vi "solar_type Get Value (ASCII).vi"(4 "Boolean as 0,1? (F)":bool, 6 "ArrayDelimiters (1D,2D)":string[](array[string]), 8 "error in (no error)":errorcluster, 9 "Use Enum Names? (F)":bool, 11 "Variant":variant) -> (0 "error out":errorcluster, 2 "Quotes Recommended?":bool, 3 "Value (ASCII)":string)   [LabVIEW 2018]
doc: "This returns the ASCII value of the variant data."
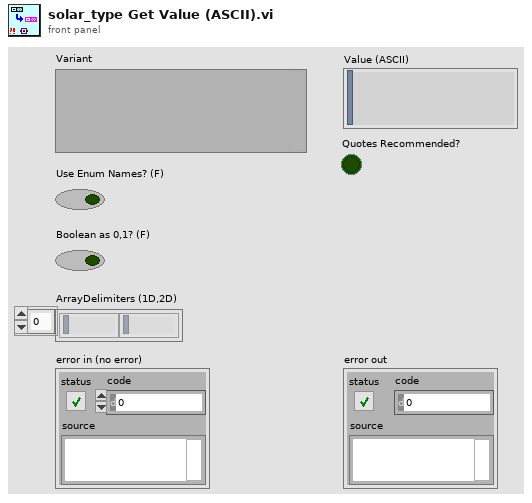
[diagram p1: front panel]
types:
  T1 = typedef "solar_type Item Type.ctl" = enum16{"NULL", "UNKNOWN", "CLUSTER", "I8", "I16", "I32", "I64", "U8", "U16", "U32", "U64", "U8_ENUM", "U16_ENUM", "U32_ENUM", "SGL", "DBL", "BOOLEAN", "STRING", "PATH", "VISA", "TAG", "TIME", "I8_1D", "I16_1D", "I32_1D", "I64_1D", "U8_1D", "U16_1D", "U32_1D", "U64_1D", "U8_ENUM_1D", "U16_ENUM_1D", "U32_ENUM_1D", "SGL_1D", "DBL_1D", "BOOLEAN_1D", "STRING_1D", "PATH_1D", "VISA_1D", "TAG_1D", "TIME_1D", "I8_2D", "I16_2D", "I32_2D", "I64_2D", "U8_2D", "U16_2D", "U32_2D", "U64_2D", "U8_ENUM_2D", "U16_ENUM_2D", "U32_ENUM_2D", "SGL_2D", "DBL_2D", "BOOLEAN_2D", "STRING_2D", "PATH_2D", "VISA_2D", "TAG_2D", "TIME_2D"}
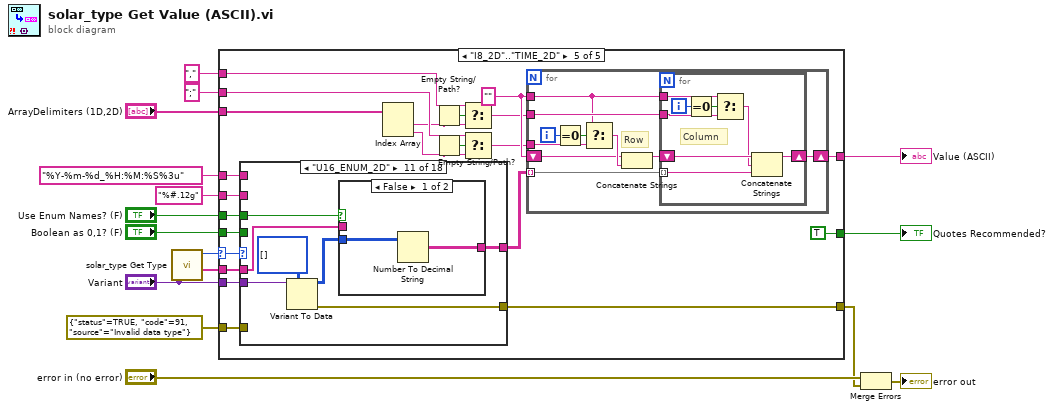
[diagram p0: block diagram]
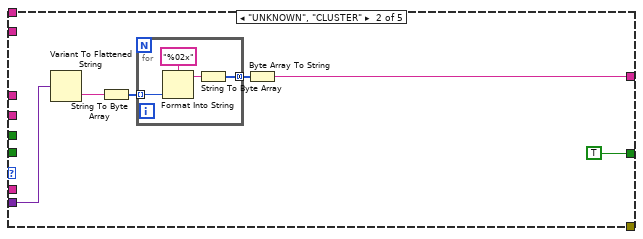
[diagram p3: hidden frame]
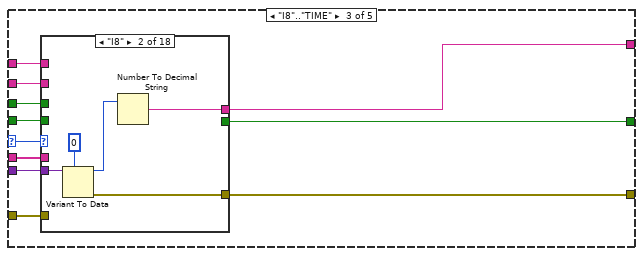
[diagram p4: hidden frame]
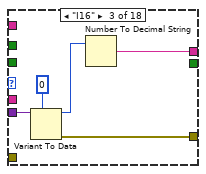
[diagram p6: hidden frame]
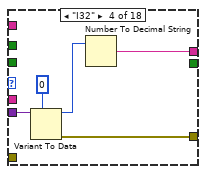
[diagram p7: hidden frame]
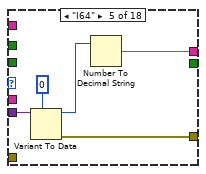
[diagram p8: hidden frame]
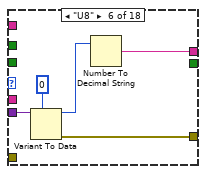
[diagram p9: hidden frame]
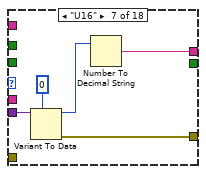
[diagram p10: hidden frame]
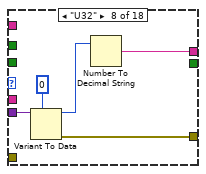
[diagram p11: hidden frame]
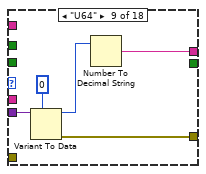
[diagram p12: hidden frame]
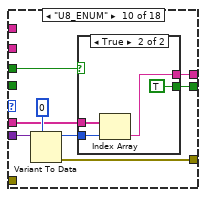
[diagram p13: hidden frame]
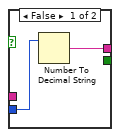
[diagram p14: hidden frame]
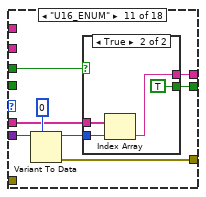
[diagram p15: hidden frame]
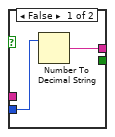
[diagram p16: hidden frame]
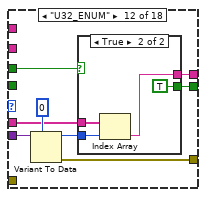
[diagram p17: hidden frame]
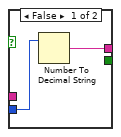
[diagram p18: hidden frame]
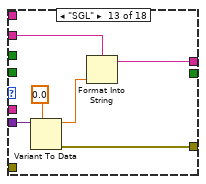
[diagram p19: hidden frame]
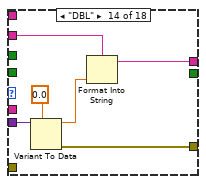
[diagram p20: hidden frame]
diagram:
  n1 = call "solar_type Get Type.vi"("Variant"="Variant") -> ("Type"=w8:T1, "Enum Names"=w2:string[])  [unwired: 4 in, 1 out]
  n2 = case shown="\"I8_2D\"..\"TIME_2D\"" w8 {
    selector: w8 -> [_ _ w36 w177 w347]
    tunnel: "Variant" -> [_ w20 w38 w178 w349]
    tunnel: [_ w21 w34 w181 w345] -> w13
    tunnel: "%Y-%m-%d_%H:%M:%S%3u" -> [_ _ w32 w173 w341]
    tunnel: [w17 _ w37 w175 w348] -> w6
    tunnel: errorcluster {"status"=TRUE, "code"=91, "source"="Invalid data type"} ("error in (no error)") -> [w17 _ w35 w179 w346]
    tunnel: "%#.12g" ("format string") -> [_ _ w33 w174 w342]
    tunnel: "," -> [_ _ _ w170 w336]
    tunnel: ";" -> [_ _ _ _ w335]
    tunnel: "Boolean as 0,1? (F)" -> [_ _ w31 w169 w334]
    tunnel: "ArrayDelimiters (1D,2D)" -> [_ _ _ w168 w333]
    tunnel: "Use Enum Names? (F)" -> [_ _ w30 w166 w330]
    tunnel: w2 -> [_ _ w29 w165 w329]
    tunnel: [_ TRUE w28 TRUE TRUE] -> w1
    frame "NULL" {
    }
    frame "UNKNOWN", "CLUSTER" {
      n3 = Variant To Flattened String(Variant=w20) -> (data string=w19:string)  [unwired: 1 out]
      n4 = String To Byte Array(string=w19) -> (unsigned byte array=w23:u8[])
      n5 = for {
        tunnel: w23 -> [w27] mode=indexing
        tunnel: [w24] -> w22 mode=concatenating
        n6 = Format Into String(format string="%02x" ("Format String"), w27) -> (resulting string=w25:string)  [unwired: 2 in, 1 out]
        n7 = String To Byte Array(string=w25) -> (unsigned byte array=w24:u8[])
      }
      n8 = Byte Array To String(unsigned byte array=w22) -> (string=w21:string)
    }
    frame "I8".."TIME" {
      n9 = case shown="\"I8\"" w36 {
        tunnel: w38 -> [_ w44 w49 w54 w59 w64 w69 w74 w79 w87 w101 w115 w127 w133 w145 w150 w156 w163]
        tunnel: [w39 w43 w48 w53 w58 w63 w68 w73 w78 w86 w100 w114 w126 w132 w144 w149 w155 w162] -> w37
        tunnel: w35 -> [w39 _ _ _ _ _ _ _ _ _ _ _ _ _ _ _ _ _]
        tunnel: [_ w40 w45 w50 w55 w60 w65 w70 w75 w83 w96 w109 w123 w129 w141 w147 w152 w159] -> w34
        tunnel: w33 -> [_ _ _ _ _ _ _ _ _ _ _ _ w122 w128 _ _ _ _]
        tunnel: w32 -> [_ _ _ _ _ _ _ _ _ _ _ _ _ _ _ _ _ w158]
        tunnel: w31 -> [_ _ _ _ _ _ _ _ _ _ _ _ _ _ w136 _ _ _]
        tunnel: w30 -> [_ _ _ _ _ _ _ _ _ w81 w95 w110 _ _ _ _ _ _]
        tunnel: w29 -> [_ _ _ _ _ _ _ _ _ w84 w98 w112 _ _ _ _ _ _]
        tunnel: [_ _ _ _ _ _ _ _ _ w80 w94 w108 _ _ _ TRUE TRUE TRUE] -> w28
        frame "NULL".."CLUSTER", "I8_1D".."TIME_2D" {
        }
        frame "I8" {
          n10 = Variant To Data(type=i8 0, Variant=w44) -> (data=w41:i8, error out=w43:errorcluster)  [unwired: 1 in]
          n11 = Number To Decimal String(number=w41) -> (decimal integer string=w40:string)  [unwired: 1 in]
        }
        frame "I16" {
          n12 = Variant To Data(type=i16 0, Variant=w49) -> (data=w46:i16, error out=w48:errorcluster)  [unwired: 1 in]
          n13 = Number To Decimal String(number=w46) -> (decimal integer string=w45:string)  [unwired: 1 in]
        }
        frame "I32" {
          n14 = Variant To Data(type=0, Variant=w54) -> (data=w51:i32, error out=w53:errorcluster)  [unwired: 1 in]
          n15 = Number To Decimal String(number=w51) -> (decimal integer string=w50:string)  [unwired: 1 in]
        }
        frame "I64" {
          n16 = Variant To Data(type=i64 0, Variant=w59) -> (data=w56:i64, error out=w58:errorcluster)  [unwired: 1 in]
          n17 = Number To Decimal String(number=w56) -> (decimal integer string=w55:string)  [unwired: 1 in]
        }
        frame "U8" {
          n18 = Variant To Data(type=u8 0, Variant=w64) -> (data=w61:u8, error out=w63:errorcluster)  [unwired: 1 in]
          n19 = Number To Decimal String(number=w61) -> (decimal integer string=w60:string)  [unwired: 1 in]
        }
        frame "U16" {
          n20 = Variant To Data(type=u16 0, Variant=w69) -> (data=w66:u16, error out=w68:errorcluster)  [unwired: 1 in]
          n21 = Number To Decimal String(number=w66) -> (decimal integer string=w65:string)  [unwired: 1 in]
        }
        frame "U32" {
          n22 = Variant To Data(type=u32 0, Variant=w74) -> (data=w71:u32, error out=w73:errorcluster)  [unwired: 1 in]
          n23 = Number To Decimal String(number=w71) -> (decimal integer string=w70:string)  [unwired: 1 in]
        }
        frame "U64" {
          n24 = Variant To Data(type=u64 0, Variant=w79) -> (data=w76:u64, error out=w78:errorcluster)  [unwired: 1 in]
          n25 = Number To Decimal String(number=w76) -> (decimal integer string=w75:string)  [unwired: 1 in]
        }
        frame "U8_ENUM" {
          n26 = Variant To Data(type=u8 0, Variant=w87) -> (data=w82:u8, error out=w86:errorcluster)  [unwired: 1 in]
          n27 = case shown="True" w81 {
            tunnel: w84 -> [_ w93]
            tunnel: [w88 w92] -> w83
            tunnel: w82 -> [w89 w91]
            tunnel: [_ TRUE] -> w80
            frame False {
              n28 = Number To Decimal String(number=w89) -> (decimal integer string=w88:string)  [unwired: 1 in]
            }
            frame True {
              n29 = Index Array(array=w93, index=w91) -> (element=w92:string)
            }
          }
        }
        frame "U16_ENUM" {
          n30 = Variant To Data(type=u16 0, Variant=w101) -> (data=w97:u16, error out=w100:errorcluster)  [unwired: 1 in]
          n31 = case shown="True" w95 {
            tunnel: w98 -> [_ w107]
            tunnel: [w102 w106] -> w96
            tunnel: w97 -> [w103 w105]
            tunnel: [_ TRUE] -> w94
            frame False {
              n32 = Number To Decimal String(number=w103) -> (decimal integer string=w102:string)  [unwired: 1 in]
            }
            frame True {
              n33 = Index Array(array=w107, index=w105) -> (element=w106:string)
            }
          }
        }
        frame "U32_ENUM" {
          n34 = Variant To Data(type=u32 0, Variant=w115) -> (data=w111:u32, error out=w114:errorcluster)  [unwired: 1 in]
          n35 = case shown="True" w110 {
            tunnel: w112 -> [_ w121]
            tunnel: [w116 w120] -> w109
            tunnel: w111 -> [w117 w119]
            tunnel: [_ TRUE] -> w108
            frame False {
              n36 = Number To Decimal String(number=w117) -> (decimal integer string=w116:string)  [unwired: 1 in]
            }
            frame True {
              n37 = Index Array(array=w121, index=w119) -> (element=w120:string)
            }
          }
        }
        frame "SGL" {
          n38 = Variant To Data(type=sgl 0.0, Variant=w127) -> (data=w124:sgl, error out=w126:errorcluster)  [unwired: 1 in]
          n39 = Format Into String(format string=w122, w124) -> (resulting string=w123:string)  [unwired: 2 in, 1 out]
        }
        frame "DBL" {
          n40 = Variant To Data(type=0.0, Variant=w133) -> (data=w130:dbl, error out=w132:errorcluster)  [unwired: 1 in]
          n41 = Format Into String(format string=w128, w130) -> (resulting string=w129:string)  [unwired: 2 in, 1 out]
        }
        frame "BOOLEAN" {
          n42 = Variant To Data(type=FALSE, Variant=w145) -> (data=w142:bool, error out=w144:errorcluster)  [unwired: 1 in]
          n43 = Select(t="1", s=w136, f="true") -> (s? t:f=w135:string)
          n44 = Select(t="0", s=w136, f="false") -> (s? t:f=w134:string)
          n45 = Select(t=w135, s=w142, f=w134) -> (s? t:f=w141:string)
        }
        frame "STRING", "VISA", "TAG" {
          n46 = Variant To Data(type="", Variant=w150) -> (data=w147:string, error out=w149:errorcluster)  [unwired: 1 in]
        }
        frame "PATH" {
          n47 = Variant To Data(type=path "", Variant=w156) -> (data=w153:path, error out=w155:errorcluster)  [unwired: 1 in]
          n48 = Path To String(path=w153) -> (string=w152:string)
        }
        frame "TIME" {
          n49 = Variant To Data(type=timestamp(0 s since 1904-01-01), Variant=w163) -> (data=w160:timestamp, error out=w162:errorcluster)  [unwired: 1 in]
          n50 = Format Date/Time String(time format string (%c)=w158, seconds (now)=w160) -> (date/time string=w159:string)  [unwired: 1 in]
        }
      }
    }
    frame "I8_1D".."TIME_1D" {
      w180 = ""
      n51 = case shown="\"U8_ENUM_1D\"" w177 {
        tunnel: w178 -> [_ w187 w192 w197 w202 w207 w212 w217 w222 w229 w244 w259 w273 w282 w297 w305 w310 w316]
        tunnel: [w182 w186 w191 w196 w201 w206 w211 w216 w221 w228 w243 w258 w272 w281 w296 w304 w309 w315] -> w175
        tunnel: w179 -> [w182 _ _ _ _ _ _ _ _ _ _ _ _ _ _ _ _ _]
        tunnel: [_ w183 w188 w193 w198 w203 w208 w213 w218 w224 w239 w254 w269 w278 w293 w302 w306 w312] -> w176
        tunnel: w174 -> [_ _ _ _ _ _ _ _ _ _ _ _ w268 w277 _ _ _ _]
        tunnel: w173 -> [_ _ _ _ _ _ _ _ _ _ _ _ _ _ _ _ _ w311]
        tunnel: w169 -> [_ _ _ _ _ _ _ _ _ _ _ _ _ _ w288 _ _ _]
        tunnel: w166 -> [_ _ _ _ _ _ _ _ _ w225 w240 w255 _ _ _ _ _ _]
        tunnel: w165 -> [_ _ _ _ _ _ _ _ _ w223 w238 w253 _ _ _ _ _ _]
        frame "NULL".."TIME", "I8_2D".."TIME_2D" {
        }
        frame "I8_1D" {
          n52 = Variant To Data(type=i8[] [], Variant=w187) -> (data=w184:i8[], error out=w186:errorcluster)  [unwired: 1 in]
          n53 = Number To Decimal String(number=w184) -> (decimal integer string=w183:string[])  [unwired: 1 in]
        }
        frame "I16_1D" {
          n54 = Variant To Data(type=i16[] [], Variant=w192) -> (data=w189:i16[], error out=w191:errorcluster)  [unwired: 1 in]
          n55 = Number To Decimal String(number=w189) -> (decimal integer string=w188:string[])  [unwired: 1 in]
        }
        frame "I32_1D" {
          n56 = Variant To Data(type=i32[] [], Variant=w197) -> (data=w194:i32[], error out=w196:errorcluster)  [unwired: 1 in]
          n57 = Number To Decimal String(number=w194) -> (decimal integer string=w193:string[])  [unwired: 1 in]
        }
        frame "I64_1D" {
          n58 = Variant To Data(type=i64[] [], Variant=w202) -> (data=w199:i64[], error out=w201:errorcluster)  [unwired: 1 in]
          n59 = Number To Decimal String(number=w199) -> (decimal integer string=w198:string[])  [unwired: 1 in]
        }
        frame "U8_1D" {
          n60 = Variant To Data(type=u8[] [], Variant=w207) -> (data=w204:u8[], error out=w206:errorcluster)  [unwired: 1 in]
          n61 = Number To Decimal String(number=w204) -> (decimal integer string=w203:string[])  [unwired: 1 in]
        }
        frame "U16_1D" {
          n62 = Variant To Data(type=u16[] [], Variant=w212) -> (data=w209:u16[], error out=w211:errorcluster)  [unwired: 1 in]
          n63 = Number To Decimal String(number=w209) -> (decimal integer string=w208:string[])  [unwired: 1 in]
        }
        frame "U32_1D" {
          n64 = Variant To Data(type=u32[] [], Variant=w217) -> (data=w214:u32[], error out=w216:errorcluster)  [unwired: 1 in]
          n65 = Number To Decimal String(number=w214) -> (decimal integer string=w213:string[])  [unwired: 1 in]
        }
        frame "U64_1D" {
          n66 = Variant To Data(type=u64[] [], Variant=w222) -> (data=w219:u64[], error out=w221:errorcluster)  [unwired: 1 in]
          n67 = Number To Decimal String(number=w219) -> (decimal integer string=w218:string[])  [unwired: 1 in]
        }
        frame "U8_ENUM_1D" {
          n68 = Variant To Data(type=u8[] [], Variant=w229) -> (data=w226:u8[], error out=w228:errorcluster)  [unwired: 1 in]
          n69 = case shown="True" w225 {
            tunnel: w223 -> [_ w234]
            tunnel: [w230 w233] -> w224
            tunnel: w226 -> [w231 w232]
            frame False {
              n70 = Number To Decimal String(number=w231) -> (decimal integer string=w230:string[])  [unwired: 1 in]
            }
            frame True {
              n71 = for {
                tunnel: w234 -> [w237]
                tunnel: [w236] -> w233 mode=indexing
                tunnel: w232 -> [w235] mode=indexing
                n72 = Index Array(array=w237, index=w235) -> (element=w236:string)
              }
            }
          }
        }
        frame "U16_ENUM_1D" {
          n73 = Variant To Data(type=u16[] [], Variant=w244) -> (data=w241:u16[], error out=w243:errorcluster)  [unwired: 1 in]
          n74 = case shown="True" w240 {
            tunnel: w238 -> [_ w249]
            tunnel: [w245 w248] -> w239
            tunnel: w241 -> [w246 w247]
            frame False {
              n75 = Number To Decimal String(number=w246) -> (decimal integer string=w245:string[])  [unwired: 1 in]
            }
            frame True {
              n76 = for {
                tunnel: w249 -> [w252]
                tunnel: [w251] -> w248 mode=indexing
                tunnel: w247 -> [w250] mode=indexing
                n77 = Index Array(array=w252, index=w250) -> (element=w251:string)
              }
            }
          }
        }
        frame "U32_ENUM_1D" {
          n78 = Variant To Data(type=u32[] [], Variant=w259) -> (data=w256:u32[], error out=w258:errorcluster)  [unwired: 1 in]
          n79 = case shown="True" w255 {
            tunnel: w253 -> [_ w264]
            tunnel: [w260 w263] -> w254
            tunnel: w256 -> [w261 w262]
            frame False {
              n80 = Number To Decimal String(number=w261) -> (decimal integer string=w260:string[])  [unwired: 1 in]
            }
            frame True {
              n81 = for {
                tunnel: w264 -> [w267]
                tunnel: [w266] -> w263 mode=indexing
                tunnel: w262 -> [w265] mode=indexing
                n82 = Index Array(array=w267, index=w265) -> (element=w266:string)
              }
            }
          }
        }
        frame "SGL_1D" {
          n83 = Variant To Data(type=sgl[] [], Variant=w273) -> (data=w270:sgl[], error out=w272:errorcluster)  [unwired: 1 in]
          n84 = for {
            tunnel: w270 -> [w276] mode=indexing
            tunnel: [w275] -> w269 mode=indexing
            tunnel: w268 -> [w274]
            n85 = Format Into String(format string=w274, w276) -> (resulting string=w275:string)  [unwired: 2 in, 1 out]
          }
        }
        frame "DBL_1D" {
          n86 = Variant To Data(type=dbl[] [], Variant=w282) -> (data=w279:dbl[], error out=w281:errorcluster)  [unwired: 1 in]
          n87 = for {
            tunnel: w279 -> [w285] mode=indexing
            tunnel: [w284] -> w278 mode=indexing
            tunnel: w277 -> [w283]
            n88 = Format Into String(format string=w283, w285) -> (resulting string=w284:string)  [unwired: 2 in, 1 out]
          }
        }
        frame "BOOLEAN_1D" {
          n89 = Variant To Data(type=bool[] [], Variant=w297) -> (data=w294:bool[], error out=w296:errorcluster)  [unwired: 1 in]
          n90 = Select(t="1", s=w288, f="true") -> (s? t:f=w287:string)
          n91 = Select(t="0", s=w288, f="false") -> (s? t:f=w286:string)
          n92 = for {
            tunnel: w294 -> [w301] mode=indexing
            tunnel: [w300] -> w293 mode=indexing
            tunnel: w287 -> [w299]
            tunnel: w286 -> [w298]
            n93 = Select(t=w299, s=w301, f=w298) -> (s? t:f=w300:string)
          }
        }
        frame "STRING_1D", "VISA_1D", "TAG_1D" {
          n94 = Variant To Data(type=string[] [], Variant=w305) -> (data=w302:string[], error out=w304:errorcluster)  [unwired: 1 in]
        }
        frame "PATH_1D" {
          n95 = Variant To Data(type=path[] [], Variant=w310) -> (data=w307:path[], error out=w309:errorcluster)  [unwired: 1 in]
          n96 = Path To String(path=w307) -> (string=w306:string[])
        }
        frame "TIME_1D" {
          n97 = Variant To Data(type=timestamp[] [], Variant=w316) -> (data=w313:timestamp[], error out=w315:errorcluster)  [unwired: 1 in]
          n98 = for {
            tunnel: w313 -> [w317] mode=indexing
            tunnel: [w319] -> w312 mode=indexing
            tunnel: w311 -> [w318]
            n99 = Format Date/Time String(time format string (%c)=w318, seconds (now)=w317) -> (date/time string=w319:string)  [unwired: 1 in]
          }
        }
      }
      n100 = Index Array(array=w168) -> (element=w167:string)  [unwired: 1 in]
      n101 = Empty String/Path?(string/path=w167) -> (empty?=w172:bool)
      n102 = Select(t=w170, s=w172, f=w167) -> (s? t:f=w171:string)
      n103 = for {
        shift-right: [w326] -> w181
        shift-left: w180 -> [w327]
        tunnel: w171 -> [w322]
        tunnel: w180 -> [w321]
        tunnel: w176 -> [w320] mode=indexing
        i -> [w325]
        # "Column"
        n104 = Equal To 0?(x=w325) -> (x = 0?=w324:bool)
        n105 = Select(t=w321, s=w324, f=w322) -> (s? t:f=w323:string)
        n106 = Concatenate Strings(w327, w323, w320) -> (w326:string)
      }
    }
    frame "I8_2D".."TIME_2D" {
      w344 = ""
      n107 = case shown="\"U16_ENUM_2D\"" w347 {
        tunnel: w349 -> [_ w355 w360 w365 w370 w375 w380 w385 w390 w397 w415 w433 w450 w462 w480 w492 w497 w503]
        tunnel: [w350 w354 w359 w364 w369 w374 w379 w384 w389 w396 w414 w432 w449 w461 w479 w491 w496 w502] -> w348
        tunnel: w346 -> [w350 _ _ _ _ _ _ _ _ _ _ _ _ _ _ _ _ _]
        tunnel: [_ w351 w356 w361 w366 w371 w376 w381 w386 w391 w409 w427 w446 w458 w477 w489 w493 w499] -> w343
        tunnel: w342 -> [_ _ _ _ _ _ _ _ _ _ _ _ w445 w457 _ _ _ _]
        tunnel: w341 -> [_ _ _ _ _ _ _ _ _ _ _ _ _ _ _ _ _ w498]
        tunnel: w334 -> [_ _ _ _ _ _ _ _ _ _ _ _ _ _ w471 _ _ _]
        tunnel: w330 -> [_ _ _ _ _ _ _ _ _ w393 w411 w429 _ _ _ _ _ _]
        tunnel: w329 -> [_ _ _ _ _ _ _ _ _ w392 w410 w428 _ _ _ _ _ _]
        frame "NULL".."TIME_1D" {
        }
        frame "I8_2D" {
          n108 = Variant To Data(type=i8[][] [], Variant=w355) -> (data=w352:i8[][], error out=w354:errorcluster)  [unwired: 1 in]
          n109 = Number To Decimal String(number=w352) -> (decimal integer string=w351:string[][])  [unwired: 1 in]
        }
        frame "I16_2D" {
          n110 = Variant To Data(type=i16[][] [], Variant=w360) -> (data=w357:i16[][], error out=w359:errorcluster)  [unwired: 1 in]
          n111 = Number To Decimal String(number=w357) -> (decimal integer string=w356:string[][])  [unwired: 1 in]
        }
        frame "I32_2D" {
          n112 = Variant To Data(type=i32[][] [], Variant=w365) -> (data=w362:i32[][], error out=w364:errorcluster)  [unwired: 1 in]
          n113 = Number To Decimal String(number=w362) -> (decimal integer string=w361:string[][])  [unwired: 1 in]
        }
        frame "I64_2D" {
          n114 = Variant To Data(type=i64[][] [], Variant=w370) -> (data=w367:i64[][], error out=w369:errorcluster)  [unwired: 1 in]
          n115 = Number To Decimal String(number=w367) -> (decimal integer string=w366:string[][])  [unwired: 1 in]
        }
        frame "U8_2D" {
          n116 = Variant To Data(type=u8[][] [], Variant=w375) -> (data=w372:u8[][], error out=w374:errorcluster)  [unwired: 1 in]
          n117 = Number To Decimal String(number=w372) -> (decimal integer string=w371:string[][])  [unwired: 1 in]
        }
        frame "U16_2D" {
          n118 = Variant To Data(type=u16[][] [], Variant=w380) -> (data=w377:u16[][], error out=w379:errorcluster)  [unwired: 1 in]
          n119 = Number To Decimal String(number=w377) -> (decimal integer string=w376:string[][])  [unwired: 1 in]
        }
        frame "U32_2D" {
          n120 = Variant To Data(type=u32[][] [], Variant=w385) -> (data=w382:u32[][], error out=w384:errorcluster)  [unwired: 1 in]
          n121 = Number To Decimal String(number=w382) -> (decimal integer string=w381:string[][])  [unwired: 1 in]
        }
        frame "U64_2D" {
          n122 = Variant To Data(type=u64[][] [], Variant=w390) -> (data=w387:u64[][], error out=w389:errorcluster)  [unwired: 1 in]
          n123 = Number To Decimal String(number=w387) -> (decimal integer string=w386:string[][])  [unwired: 1 in]
        }
        frame "U8_ENUM_2D" {
          n124 = Variant To Data(type=u8[][] [], Variant=w397) -> (data=w394:u8[][], error out=w396:errorcluster)  [unwired: 1 in]
          n125 = case shown="False" w393 {
            tunnel: w392 -> [_ w402]
            tunnel: [w398 w401] -> w391
            tunnel: w394 -> [w399 w400]
            frame False {
              n126 = Number To Decimal String(number=w399) -> (decimal integer string=w398:string[][])  [unwired: 1 in]
            }
            frame True {
              n127 = for {
                tunnel: w402 -> [w405]
                tunnel: [w404] -> w401 mode=indexing
                tunnel: w400 -> [w403] mode=indexing
                n128 = for {
                  tunnel: w405 -> [w408]
                  tunnel: [w407] -> w404 mode=indexing
                  tunnel: w403 -> [w406] mode=indexing
                  n129 = Index Array(array=w408, index=w406) -> (element=w407:string)
                }
              }
            }
          }
        }
        frame "U16_ENUM_2D" {
          n130 = Variant To Data(type=u16[][] [], Variant=w415) -> (data=w412:u16[][], error out=w414:errorcluster)  [unwired: 1 in]
          n131 = case shown="False" w411 {
            tunnel: w410 -> [_ w420]
            tunnel: [w416 w419] -> w409
            tunnel: w412 -> [w417 w418]
            frame False {
              n132 = Number To Decimal String(number=w417) -> (decimal integer string=w416:string[][])  [unwired: 1 in]
            }
            frame True {
              n133 = for {
                tunnel: w420 -> [w423]
                tunnel: [w422] -> w419 mode=indexing
                tunnel: w418 -> [w421] mode=indexing
                n134 = for {
                  tunnel: w423 -> [w426]
                  tunnel: [w425] -> w422 mode=indexing
                  tunnel: w421 -> [w424] mode=indexing
                  n135 = Index Array(array=w426, index=w424) -> (element=w425:string)
                }
              }
            }
          }
        }
        frame "U32_ENUM_2D" {
          n136 = Variant To Data(type=u32[][] [], Variant=w433) -> (data=w430:u32[][], error out=w432:errorcluster)  [unwired: 1 in]
          n137 = case shown="False" w429 {
            tunnel: w428 -> [_ w438]
            tunnel: [w434 w437] -> w427
            tunnel: w430 -> [w435 w436]
            frame False {
              n138 = Number To Decimal String(number=w435) -> (decimal integer string=w434:string[][])  [unwired: 1 in]
            }
            frame True {
              n139 = for {
                tunnel: w438 -> [w441]
                tunnel: [w440] -> w437 mode=indexing
                tunnel: w436 -> [w439] mode=indexing
                n140 = for {
                  tunnel: w441 -> [w444]
                  tunnel: [w443] -> w440 mode=indexing
                  tunnel: w439 -> [w442] mode=indexing
                  n141 = Index Array(array=w444, index=w442) -> (element=w443:string)
                }
              }
            }
          }
        }
        frame "SGL_2D" {
          n142 = Variant To Data(type=sgl[][] [], Variant=w450) -> (data=w447:sgl[][], error out=w449:errorcluster)  [unwired: 1 in]
          n143 = for {
            tunnel: w447 -> [w453] mode=indexing
            tunnel: [w452] -> w446 mode=indexing
            tunnel: w445 -> [w451]
            n144 = for {
              tunnel: w453 -> [w456] mode=indexing
              tunnel: [w455] -> w452 mode=indexing
              tunnel: w451 -> [w454]
              n145 = Format Into String(format string=w454, w456) -> (resulting string=w455:string)  [unwired: 2 in, 1 out]
            }
          }
        }
        frame "DBL_2D" {
          n146 = Variant To Data(type=dbl[][] [], Variant=w462) -> (data=w459:dbl[][], error out=w461:errorcluster)  [unwired: 1 in]
          n147 = for {
            tunnel: w459 -> [w465] mode=indexing
            tunnel: [w464] -> w458 mode=indexing
            tunnel: w457 -> [w463]
            n148 = for {
              tunnel: w465 -> [w468] mode=indexing
              tunnel: [w467] -> w464 mode=indexing
              tunnel: w463 -> [w466]
              n149 = Format Into String(format string=w466, w468) -> (resulting string=w467:string)  [unwired: 2 in, 1 out]
            }
          }
        }
        frame "BOOLEAN_2D" {
          n150 = Variant To Data(type=bool[][] [], Variant=w480) -> (data=w476:bool[][], error out=w479:errorcluster)  [unwired: 1 in]
          n151 = Select(t="1", s=w471, f="true") -> (s? t:f=w470:string)
          n152 = Select(t="0", s=w471, f="false") -> (s? t:f=w469:string)
          n153 = for {
            tunnel: [w484] -> w477 mode=indexing
            tunnel: w476 -> [w483] mode=indexing
            tunnel: w470 -> [w482]
            tunnel: w469 -> [w481]
            n154 = for {
              tunnel: w483 -> [w488] mode=indexing
              tunnel: [w487] -> w484 mode=indexing
              tunnel: w482 -> [w486]
              tunnel: w481 -> [w485]
              n155 = Select(t=w486, s=w488, f=w485) -> (s? t:f=w487:string)
            }
          }
        }
        frame "STRING_2D", "VISA_2D", "TAG_2D" {
          n156 = Variant To Data(type=string[][] [], Variant=w492) -> (data=w489:string[][], error out=w491:errorcluster)  [unwired: 1 in]
        }
        frame "PATH_2D" {
          n157 = Variant To Data(type=path[][] [], Variant=w497) -> (data=w494:path[][], error out=w496:errorcluster)  [unwired: 1 in]
          n158 = Path To String(path=w494) -> (string=w493:string[][])
        }
        frame "TIME_2D" {
          n159 = Variant To Data(type=timestamp[][] [], Variant=w503) -> (data=w500:timestamp[][], error out=w502:errorcluster)  [unwired: 1 in]
          n160 = for {
            tunnel: w500 -> [w506] mode=indexing
            tunnel: [w505] -> w499 mode=indexing
            tunnel: w498 -> [w504]
            n161 = for {
              tunnel: w506 -> [w507] mode=indexing
              tunnel: [w509] -> w505 mode=indexing
              tunnel: w504 -> [w508]
              n162 = Format Date/Time String(time format string (%c)=w508, seconds (now)=w507) -> (date/time string=w509:string)  [unwired: 1 in]
            }
          }
        }
      }
      n163 = Index Array(array=w333) -> (element #1=w332:string, element #2=w331:string)  [unwired: 2 in]
      n164 = Empty String/Path?(string/path=w332) -> (empty?=w340:bool)
      n165 = Empty String/Path?(string/path=w331) -> (empty?=w339:bool)
      n166 = Select(t=w336, s=w340, f=w332) -> (s? t:f=w338:string)
      n167 = Select(t=w335, s=w339, f=w331) -> (s? t:f=w337:string)
      n168 = for {
        shift-right: [w512] -> w345
        shift-left: w344 -> [w515]
        tunnel: w338 -> [w518]
        tunnel: w337 -> [w513]
        tunnel: w344 -> [w511]
        tunnel: w343 -> [w510] mode=indexing
        i -> [w517]
        # "Row"
        n169 = Equal To 0?(x=w517) -> (x = 0?=w519:bool)
        n170 = Select(t=w511, s=w519, f=w513) -> (s? t:f=w516:string)
        n171 = Concatenate Strings(w515, w516) -> (w514:string)
        n172 = for {
          shift-right: [w526] -> w512
          shift-left: w514 -> [w527]
          tunnel: w518 -> [w522]
          tunnel: w511 -> [w521]
          tunnel: w510 -> [w520] mode=indexing
          i -> [w525]
          # "Column"
          n173 = Equal To 0?(x=w525) -> (x = 0?=w524:bool)
          n174 = Select(t=w521, s=w524, f=w522) -> (s? t:f=w523:string)
          n175 = Concatenate Strings(w527, w523, w520) -> (w526:string)
        }
      }
    }
  }
  "Value (ASCII)" <- w13
  "Quotes Recommended?" <- w1
  n176 = Merge Errors("error in (no error)", w6) -> (→"error out":errorcluster)
